vi "MAP_DIM.vi"() -> (0 "MAP_DIM":i16=64)   [LabVIEW 2020]
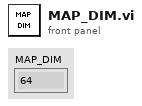
[diagram p1: front panel]
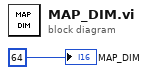
[diagram p0: block diagram]
diagram:
  "MAP_DIM" <- i16 64
